vi "clearpath_set_reset.vi"(0 "ClearpathComm":T1) -> ()   [LabVIEW 2012, in "clearpath_interface.lvlib"]
doc: "Formats a Reset Processor command (0x2000) to reset the microcontroller. A reset should not affect auxiliary sensor power (including the bus the cRIO is powered from). Uses the onboard Clearpath library to perform the actual message formatting."
uses:
  clearpath_interface.lvlib
  cwrap_crio.dll
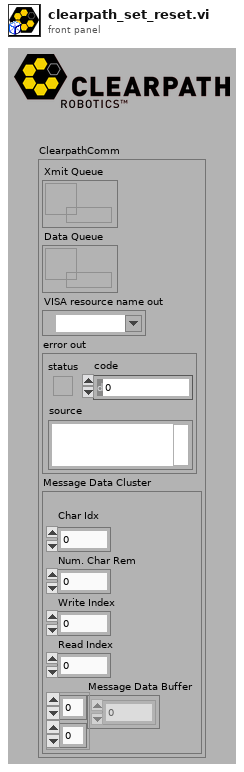
[diagram p1: front panel]
types:
  T1 = cluster{"Xmit Queue":refnum<queue>, "Data Queue":refnum<queue>, "VISA resource name out":refnum<visa-resource-name>, "error out":errorcluster, "Message Data Cluster":cluster{"\nChar Idx":u8, "Num. Char Rem":u8, "Write Index":u8, "Read Index":u8, "Message Data Buffer":u8[][]}}
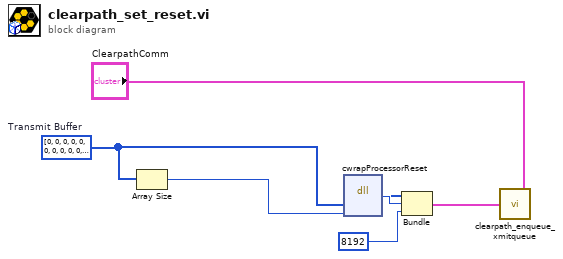
[diagram p0: block diagram]
diagram:
  w1 = u8[] [0, 0, 0, 0, 0, 0, 0, 0, 0, 0, 0, 0, 0, 0, 0, 0, 0, 0, 0, 0, 0, 0, 0, 0, 0, 0, 0, 0, 0, 0, 1, 0, 0, 0, 5]  # Transmit Buffer
  n1 = Array Size(array=w1) -> (size(s)=w5:i32)
  n2 = dll-call lib="C:/Users/tebbeam/Documents/GitHub/IGVC-2013/Code/Project 1.0/Motors/Husky/cwrap_cRIO.*" fn="cwrapProcessorReset"("buf"=w1, "buf_size"=w5) -> ("return type"=w7:i32, "buf"=w6:u8[])  [unwired: 4 in, 2 out]
  n3 = Bundle("buf"=w6, "return type"=w7, 8192) -> (w3:cluster{"buf":u8[], "return type":i32, i32})  [unwired: 1 in]
  n4 = call "clearpath_enqueue_xmitqueue.vi"("ClearpathComm"="ClearpathComm", "Cluster"=w3) -> ()
